vi "new.vi"(8 "Error In":errorcluster, 10 "ref":refnum<vi>, 11 "GObject in":refnum<class "GObject.lvclass">) -> (0 "Error Out":errorcluster, 3 "GObject out":refnum<class "GObject.lvclass">)   [LabVIEW 2023, in "TLC_Scripto.lvlib" / "GObject.lvclass"]
uses:
  GObject.lvclass
  GObject.lvclass/GObject.ctl
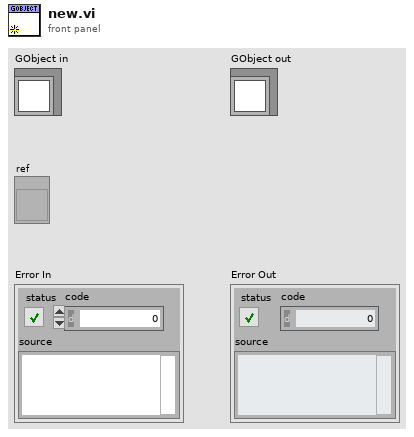
[diagram p1: front panel]
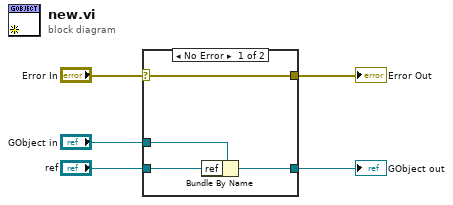
[diagram p0: block diagram]
diagram:
  n1 = case shown="No Error" "Error In" {
    selector: "Error In" -> [w7 w10]
    tunnel: "GObject in" -> [w9 w11]
    tunnel: [w8 w11] -> w5
    tunnel: [w7 w10] -> w3
    tunnel: "ref" -> [w6 _]
    frame No Error {
      n2 = Bundle By Name(cluster=w9, "ref"=w6) -> (w8:refnum<class "GObject.lvclass">)
    }
    frame Error {
    }
  }
  "GObject out" <- w5
  "Error Out" <- w3
